vi "AK TCP Factory.vi"(8 "error in (no error)":errorcluster, 10 "settings":T1) -> (0 "error out":errorcluster, 3 "protocol out":refnum<class "Protocol Parent.lvclass">)   [LabVIEW 2019, in "Instrument Addon Scripting API.lvlib"]
doc: "Instantiates a new AK TCP Protocol object using the provided AK TCP settings."
uses:
  Instrument Addon Scripting API.lvlib
  Includes/Protocols.lvlibp/AK TCP/AK TCP Settings.ctl
  Includes/Protocols.lvlibp/Protocol Parent/Protocol Parent.lvclass
  Includes/Protocols.lvlibp/AK TCP/AK TCP.lvclass
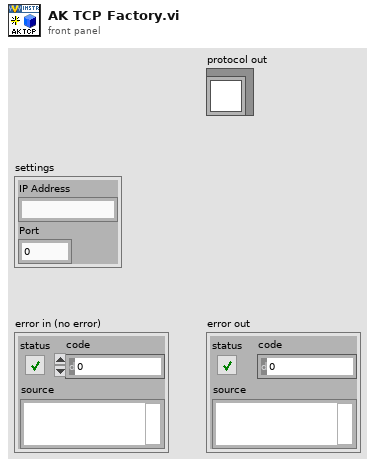
[diagram p1: front panel]
types:
  T1 = typedef "Protocols.lvlibp/AK TCP.lvclass/AK TCP Settings.ctl" = cluster{"IP Address":string, "Port":u16}
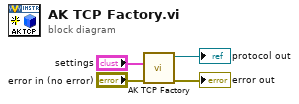
[diagram p0: block diagram]
diagram:
  n1 = call "AK TCP Factory.vi"("error in (no error)"="error in (no error)", "AK TCP settings"="settings") -> ("error out"=→"error out":errorcluster, "protocol out"=→"protocol out":refnum<class "Protocol Parent.lvclass">)  [unwired: 8 in]
